vi "ProdaNG.Example.GetTestSteps2.vi"() -> ()   [LabVIEW 2015]
uses:
  Controls/ProdaNG.Identification.ctl
  Controls/ProdaNG.TestStep.ctl
  Controls/ProdaNG.ProcessStep.ctl
  Controls/ProdaNG.Process.ctl
  Controls/ProdaNG.ProcessStepParam.ctl
  <vilib>/Utility/miscctls.llb/LVRowAndColumnUnsignedTypeDef.ctl
panel:
  in  "ResultStatus":i32(listbox)
  out "Identification":T1
  in  "ButtonUpdate":bool
  in  "ButtonRead":bool
  in  "Results":i32(listbox)
  out "ProcStepParams":T2[](array[typedef])
  out "Process":T3
  out "ProcStep":T4[](array[typedef])
  out "TestSteps":T5[](array[typedef])
  in  "Product Serial Number":string="1160131100027"
  out "ID":T6
  in  "System":string="lin"
  in  "Wabco Number":string="0000001230"
  in  "Connection string":string="lcptb/lcptb@WCQPRO"
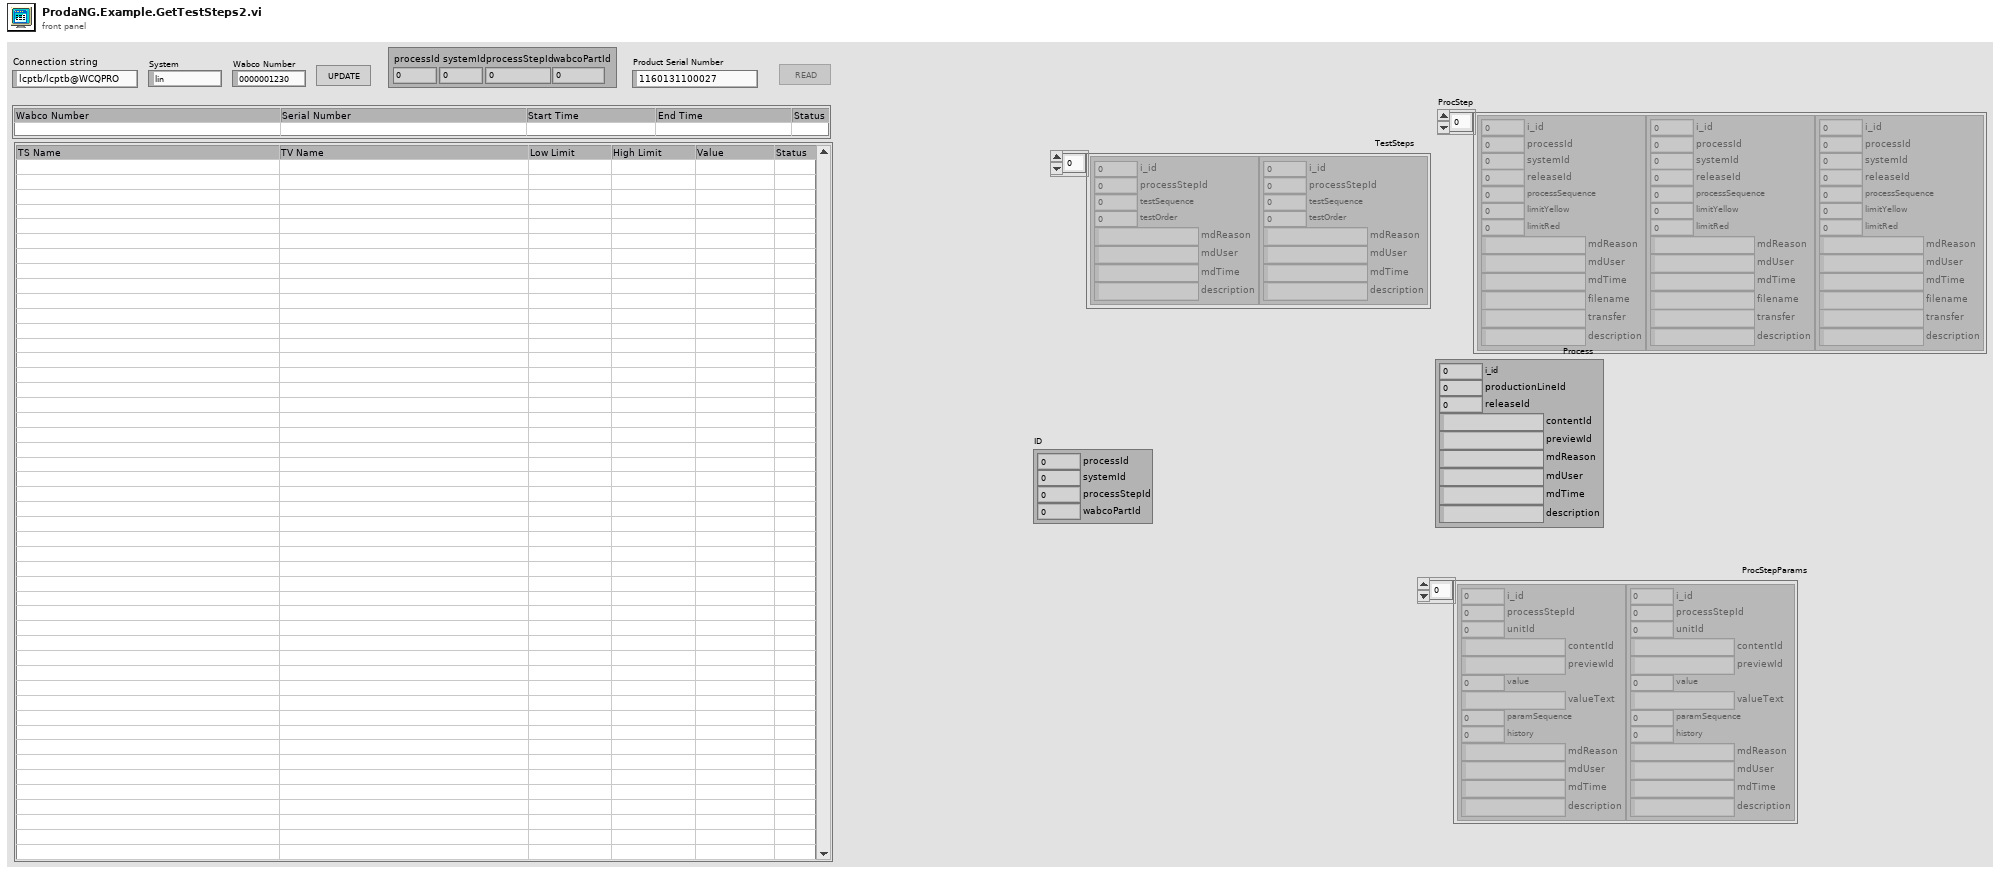
[diagram p1: front panel]
types:
  T1 = cluster{"processId":i32, "systemId":i32, "processStepId":i32, "wabcoPartId":i32}
  T2 = typedef "ProdaNG.ProcessStepParam.ctl" = cluster{"i_id":i32, "processStepId":i32, "unitId":i32, "contentId":string, "previewId":string, "value":dbl, "valueText":string, "paramSequence":i32, "history":i32, "mdReason":string, "mdUser":string, "mdTime":string, "description":string}
  T3 = typedef "ProdaNG.Process.ctl" = cluster{"i_id":i32, "productionLineId":i32, "releaseId":i32, "contentId":string, "previewId":string, "mdReason":string, "mdUser":string, "mdTime":string, "description":string}
  T4 = typedef "ProdaNG.ProcessStep.ctl" = cluster{"i_id":i32, "processId":i32, "systemId":i32, "releaseId":i32, "processSequence":i32, "limitYellow":dbl, "limitRed":dbl, "mdReason":string, "mdUser":string, "mdTime":string, "filename":string, "transfer":string, "description":string}
  T5 = typedef "ProdaNG.TestStep.ctl" = cluster{"i_id":i32, "processStepId":i32, "testSequence":i32, "testOrder":i32, "mdReason":string, "mdUser":string, "mdTime":string, "description":string}
  T6 = typedef "ProdaNG.Identification.ctl" = cluster{"processId":i32, "systemId":i32, "processStepId":i32, "wabcoPartId":i32}
  T7 = enum8{"Enabled", "Disabled", "Disabled and Grayed Out"}
  T8 = typedef "LVRowAndColumnUnsignedTypeDef.ctl" = cluster{"Row":u32, "Column":u32}
  T9 = typedef "ProdaNG.Product.ctl" = cluster{"c_id":string, "wabcoPartId":i32, "serialNumber":string, "comment":string, "individual":i32, "crProcessStepId":i32, "mdProcessStepId":i32, "crTime":string, "mdTime":string}
  T10 = typedef "ProdaNG.ProcessResult.ctl" = cluster{"c_id":string, "productId":string, "processId":i32, "statusId":i32, "startTime":string, "endTime":string}
  T11 = typedef "ProdaNG.ProcessStepResult.ctl" = cluster{"c_id":string, "processResultId":string, "processStepId":i32, "statusId":i32, "operatorId":i32, "startTime":string, "endTime":string}
  T12 = typedef "ProdaNG.TestStepResult.ctl" = cluster{"c_id":string, "processStepResultId":string, "testStepId":i32, "statusId":i32}
  T13 = typedef "ProdaNG.TestValue.ctl" = cluster{"i_id":i32, "testStepId":i32, "releaseId":i32, "unitId":i32, "contentId":string, "previewId":string, "maximum":dbl, "minimum":dbl, "valueText":string, "testValueSequence":i32, "history":i32, "mdReason":string, "mdUser":string, "mdTime":string, "description":string}
  T14 = typedef "ProdaNG.TestValueResult.ctl" = cluster{"c_id":string, "testStepResultId":string, "testValueId":i32, "result":dbl, "statusId":i32, "contentId":string}
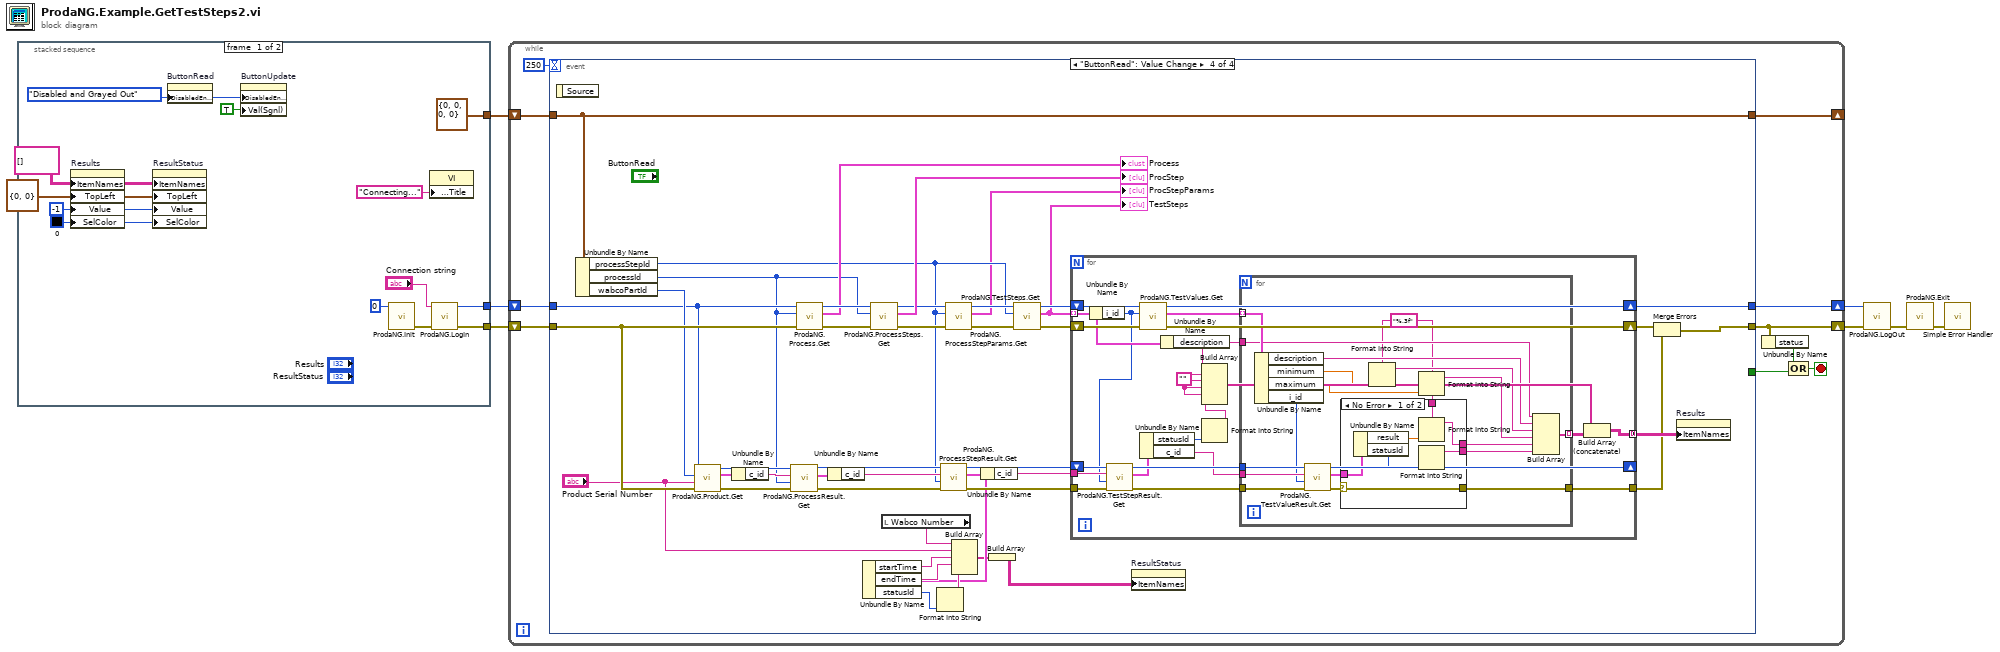
[diagram p0: block diagram]
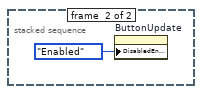
[diagram p2: hidden frame]
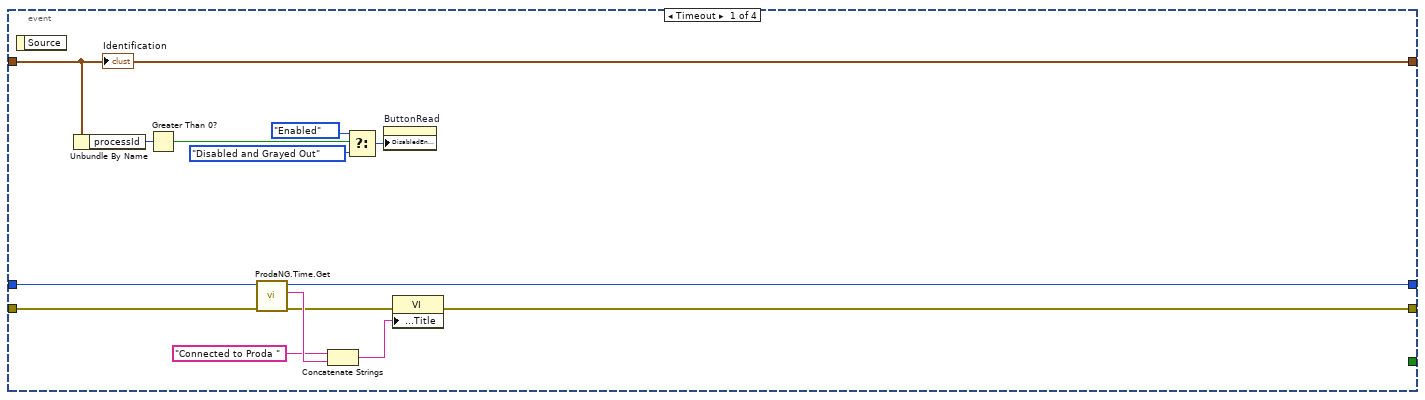
[diagram p3: hidden frame]
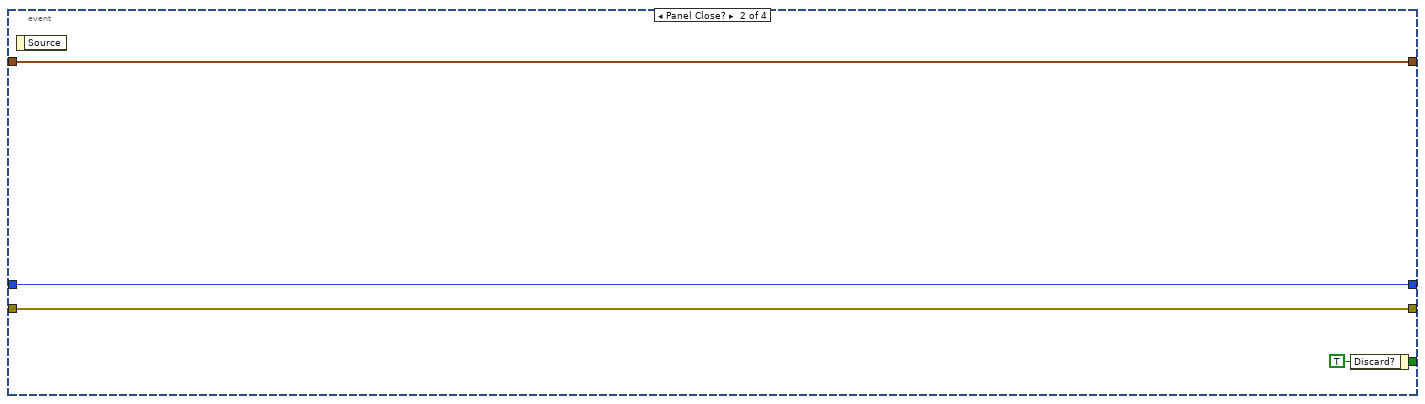
[diagram p4: hidden frame]
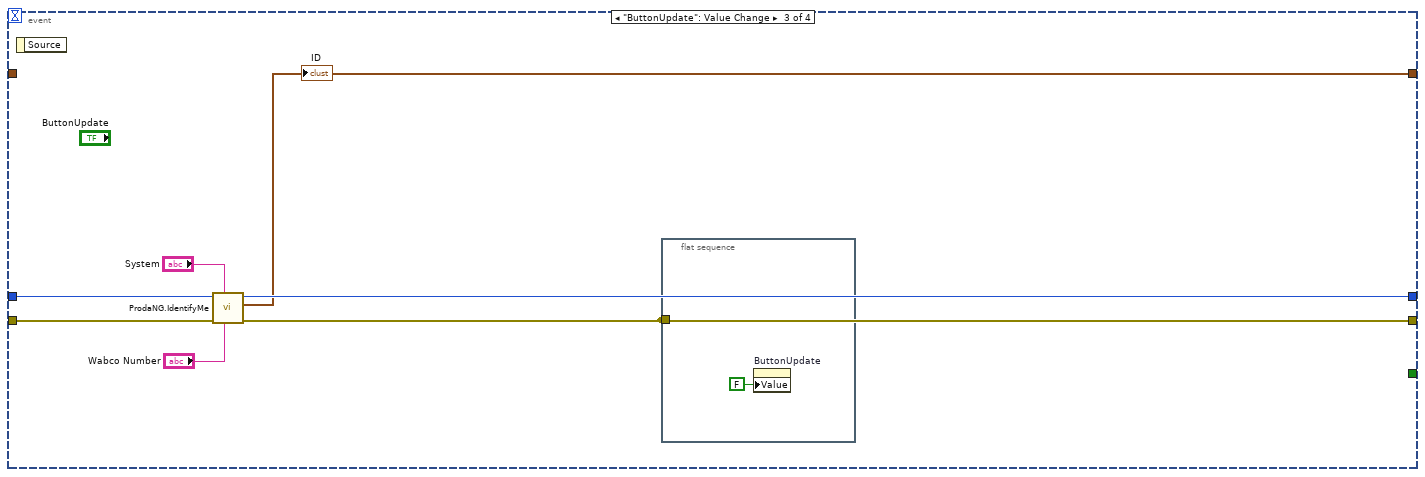
[diagram p5: hidden frame]
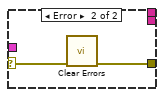
[diagram p6: hidden frame]
diagram:
  n1 = stacked-sequence {
    tunnel: [w17 _] -> w4
    tunnel: [w16 _] -> w3
    tunnel: [T6 {"processId"=0, "systemId"=0, "processStepId"=0, "wabcoPartId"=0} ("Identification") _] -> w2
    frame #0 {
      w14 = T7."Disabled and Grayed Out" ("Disabled")
      w10 = u32 0
      w9 = -1 ("Results")
      w11 = T8 {"Row"=0, "Column"=0} ("Top Left Visible Cell")
      w12 = string[][] [] ("Item Names")
      n2 = property on="Results" class="MCListbox (strict)"("ItemNames"=w12, "TopLeft"=w11, "Value"=w9, "SelColor"=w10) -> ()  [unwired: 2 in, 2 out]
      n3 = property on="ResultStatus" class="MCListbox (strict)"("ItemNames"=w12, "TopLeft"=w11, "Value"=w9, "SelColor"=w10) -> ()  [unwired: 2 in, 2 out]
      n4 = property on="ButtonRead" class="Bool"("DisabledEnum"=w14) -> ()  [unwired: 2 in, 2 out]
      n5 = property on="ButtonUpdate" class="Bool (strict)"("DisabledEnum"=w14, "Val(Sgnl)"=TRUE ("Value (Signaling)")) -> ()  [unwired: 2 in, 2 out]
      n6 = call "ProdaNG.Init.vi"("numContexts (0: unlimited)"=0 ("numContexts")) -> ("error out"=w20:errorcluster)  [unwired: 10 in]
      n7 = property class="VI"("Front Panel.Title"="Connecting..." ("Front Panel Window:Title")) -> ()  [unwired: 2 in, 2 out]
      n8 = call "ProdaNG.LogIn.vi"("error in"=w20, "ConnectionString"="Connection string") -> ("error out"=w16:errorcluster, "dbHandle"=w17:i32)  [unwired: 7 in, 1 out]
    }
    frame #1 {
      n9 = property on="ButtonUpdate" class="Bool (strict)"("DisabledEnum"=T7."Enabled" ("Disabled")) -> ()  [unwired: 2 in, 2 out]
    }
  }
  n10 = while {
    shift-right: [w25] -> w5
    shift-left: w3 -> [w30]
    shift-right: [w31] -> w6
    shift-left: w4 -> [w29]
    shift-right: [w27] -> _
    shift-left: w2 -> [w26]
    stop <- w22 stop-if-true
    n11 = event shown="[3] \"ButtonRead\": Value Change" {
      selector: _ -> [_ _ _ _]
      dyn-events: _ -> [_ _ _ _]
      timeout: 250 -> [_ _ _ _]
      tunnel: [w43 w46 w54 w89] -> w31
      tunnel: w30 -> [w44 w47 w55 w87]
      tunnel: w29 -> [w45 w46 w56 w81]
      tunnel: [w32 w47 w50 w73] -> w25
      tunnel: [w37 w49 w53 w67] -> w27
      tunnel: w26 -> [w37 w49 _ w67]
      tunnel: [_ w48 _ _] -> w24
      event Timeout {
        n12 = event-data() -> ()  [unwired: 1 in, 1 out]
        n13 = Unbundle By Name(w37) -> ("processId"=w42:i32)
        n14 = Greater Than 0?(x=w42) -> (x > 0?=w41:bool)
        n15 = call "ProdaNG.Time.Get.vi"("error in"=w44, "dbHandleIn"=w45) -> ("error out"=w33:errorcluster, "timeStr"=w36:string, "dbHandle"=w43:i32)  [unwired: 5 in, 1 out]
        n16 = Concatenate Strings("Connected to Proda " ("string"), w36) -> (w35:string)
        n17 = Select(t=T7."Enabled" ("Disabled"), s=w41, f=T7."Disabled and Grayed Out" ("Disabled")) -> (s? t:f=w40:T7)
        n18 = property on="ButtonRead" class="Bool"("DisabledEnum"=w40) -> ()  [unwired: 2 in, 2 out]
        n19 = property class="VI"(error in=w33, "Front Panel.Title"=w35) -> (error out=w32:errorcluster)  [unwired: 1 in, 1 out]
        "Identification" <- w37
      }
      event Panel Close? {
        w48 = TRUE ("Discard?")
        n20 = event-data() -> ()  [unwired: 1 in, 1 out]
        n21 = event-data("Discard?"=w48) -> ()  [unwired: 1 in, 1 out]
      }
      event "ButtonUpdate": Value Change {
        n22 = event-data() -> ()  [unwired: 1 in, 1 out]
        n23 = call "ProdaNG.IdentifyMe.vi"("wabcoNumber"="Wabco Number", "systemName"="System", "error in"=w55, "dbHandleIn"=w56) -> ("error out"=w50:errorcluster, "Identification"=w53:T6, "dbHandle"=w54:i32)  [unwired: 5 in]
        "ID" <- w53
        n24 = flat-sequence {
          tunnel: w50 -> [_]
          frame #0 {
            n25 = property on="ButtonUpdate" class="Bool (strict)"("Value"=FALSE ("ButtonUpdate")) -> ()  [unwired: 2 in, 2 out]
          }
        }
      }
      event "ButtonRead": Value Change {
        n26 = event-data() -> ()  [unwired: 1 in, 1 out]
        n27 = Unbundle By Name(w67) -> ("processStepId"=w76:i32, "processId"=w80:i32, "wabcoPartId"=w86:i32)
        n28 = call "ProdaNG.Product.Get.vi"("error in (no error)"=w87, "serialNumber"="Product Serial Number", "wabcoPartId"=w86, "dbHandle"=w81) -> ("error out"=w85:errorcluster, "Product"=w83:T9, "dbHandle out"=w82:i32)  [unwired: 4 in, 1 out]
        n29 = Unbundle By Name(w83) -> ("c_id"=w84:string)
        n30 = call "ProdaNG.ProcessResult.Get.vi"("error in (no error)"=w85, "processId"=w80, "productId"=w84, "dbHandle"=w82) -> ("error out"=w77:errorcluster, "ProcessResult"=w71:T10, "dbHandle out"=w78:i32)  [unwired: 4 in, 1 out]
        n31 = call "ProdaNG.Process.Get.vi"("error in (no error)"=w87, "processId"=w80, "dbHandleIn"=w81) -> ("error out"=w99:errorcluster, "Process"=→"Process":T3, "dbHandle"=w98:i32)  [unwired: 5 in, 1 out]
        n32 = Unbundle By Name(w71) -> ("c_id"=w79:string)
        n33 = call "ProdaNG.ProcessSteps.Get.vi"("error in (no error)"=w99, "processId"=w80, "dbHandleIn"=w98) -> ("error out"=w95:errorcluster, "ProcSteps"=→"ProcStep":T4[], "dbHandle"=w96:i32)  [unwired: 6 in]
        n34 = local read "Wabco Number"() -> (w58:string)
        n35 = call "ProdaNG.ProcessStepResult.Get.vi"("error in (no error)"=w77, "processStepId"=w76, "processResultId"=w79, "dbHandle"=w78) -> ("error out"=w75:errorcluster, "ProcessStepResult"=w61:T11, "dbHandle out"=w74:i32)  [unwired: 4 in, 1 out]
        n36 = Unbundle By Name(w61) -> ("startTime"=w65:string, "endTime"=w64:string, "statusId"=w63:i32)
        n37 = Format Into String(w63) -> (resulting string=w62:string)  [unwired: 3 in, 1 out]
        n38 = call "ProdaNG.ProcessStepParams.Get.vi"("error in (no error)"=w95, "processStepId"=w76, "dbHandleIn"=w96) -> ("error out"=w94:errorcluster, "ProcStepParams"=→"ProcStepParams":T2[], "dbHandle"=w93:i32)  [unwired: 6 in]
        n39 = Build Array(w58, "Product Serial Number", w65, w64, w62) -> (w60:string[])
        n40 = Unbundle By Name(w61) -> ("c_id"=w72:string)
        n41 = Build Array(w60) -> (w59:string[][])
        n42 = call "ProdaNG.TestSteps.Get.vi"("error in (no error)"=w94, "processStepId"=w76, "dbHandleIn"=w93) -> ("error out"=w91:errorcluster, "TestSteps"=w90:T5[], "dbHandle"=w92:i32)  [unwired: 6 in]
        "TestSteps" <- w90
        n43 = for {
          tunnel: w90 -> [w113] mode=indexing
          shift-right: [w120] -> w89
          shift-left: w92 -> [w121]
          shift-right: [w119] -> w88
          shift-left: w91 -> [w122]
          shift-right: [w116] -> _
          shift-left: w74 -> [w118]
          tunnel: w72 -> [w117]
          tunnel: [w105] -> w70 mode=concatenating
          tunnel: w75 -> [w110]
          tunnel: [w112] -> w68
          w106 = ""
          n44 = Unbundle By Name(w113) -> ("i_id"=w102:i32)
          n45 = call "ProdaNG.TestStepResult.Get.vi"("error in (no error)"=w110, "testStepId"=w102, "processStepResulttId"=w117, "dbHandle"=w118) -> ("error out"=w111:errorcluster, "TestStepResult"=w101:T12, "dbHandle out"=w116:i32)  [unwired: 4 in, 1 out]
          n46 = call "ProdaNG.TestValues.Get.vi"("error in (no error)"=w122, "testStepId"=w102, "dbHandleIn"=w121) -> ("error out"=w119:errorcluster, "TestStepValues"=w115:T13[], "dbHandle"=w120:i32)  [unwired: 6 in]
          n47 = Unbundle By Name(w101) -> ("statusId"=w108:i32, "c_id"=w103:string)
          n48 = Unbundle By Name(w113) -> ("description"=w109:string)
          n49 = Format Into String(w108) -> (resulting string=w107:string)  [unwired: 3 in, 1 out]
          n50 = Build Array(w109, w106, w106, w106, w106, w107) -> (w104:string[])
          n51 = for {
            tunnel: w103 -> [w140]
            tunnel: w116 -> [w139]
            tunnel: w111 -> [w138]
            tunnel: w115 -> [w137] mode=indexing
            tunnel: [w133] -> w114 mode=indexing
            tunnel: w109 -> [w130]
            tunnel: [w128] -> w112
            w123 = "%.3f" ("format string")
            n52 = Unbundle By Name(w137) -> ("description"=w131:string, "minimum"=w127:dbl, "maximum"=w124:dbl, "i_id"=w136:i32)
            n53 = call "ProdaNG.TestValueResult.Get.vi"("error in (no error)"=w138, "testValueId"=w136, "testStepResultId"=w140, "dbHandle"=w139) -> ("error out"=w129:errorcluster, "TestValueResult"=w135:T14)  [unwired: 5 in, 1 out]
            n54 = case shown="No Error" w129 {
              selector: w129 -> [w142 w149]
              tunnel: w135 -> [w147 _]
              tunnel: [w145 _] -> w134
              tunnel: [w144 _] -> w132
              tunnel: [w142 w148] -> w128
              tunnel: w123 -> [w141 _]
              frame No Error {
                n55 = Unbundle By Name(w147) -> ("result"=w146:dbl, "statusId"=w143:i32)
                n56 = Format Into String(format string=w141, w146) -> (resulting string=w144:string)  [unwired: 2 in, 1 out]
                n57 = Format Into String(w143) -> (resulting string=w145:string)  [unwired: 3 in, 1 out]
              }
              frame Error {
                n58 = call <vilib>:"Clear Errors.vi"("error in (no error)"=w149) -> ("error out"=w148:errorcluster)  [unwired: 5 in, 1 out]
              }
            }
            n59 = Format Into String(format string=w123, w127) -> (resulting string=w125:string)  [unwired: 2 in, 1 out]
            n60 = Format Into String(format string=w123, w124) -> (resulting string=w126:string)  [unwired: 2 in, 1 out]
            n61 = Build Array(w130, w131, w125, w126, w132, w134) -> (w133:string[])
          }
          n62 = Build Array (concatenate)(w104, w114) -> (w105:string[][])
        }
        n63 = property on="ResultStatus" class="MCListbox (strict)"("ItemNames"=w59) -> ()  [unwired: 2 in, 2 out]
        n64 = Merge Errors(w88, w68) -> (w73:errorcluster)
        n65 = property on="Results" class="MCListbox (strict)"("ItemNames"=w70) -> ()  [unwired: 2 in, 2 out]
      }
    }
    n66 = Unbundle By Name(w25) -> ("status"=w23:bool)
    n67 = Compound Arithmetic op=OR(w23, w24) -> (w22:bool)
  }
  n68 = call "ProdaNG.LogOut.vi"("error in"=w5, "dbHandleIn"=w6) -> ("error out"=w7:errorcluster)  [unwired: 9 in]
  n69 = call "ProdaNG.Exit.vi"("error in (no error)"=w7) -> ("error out"=w1:errorcluster)  [unwired: 10 in]
  n70 = call <vilib>:"Simple Error Handler.vi"("error in (no error)"=w1) -> ()  [unwired: 4 in, 5 out]
